vi "ATS_Buffer_to_Channel.vi"(8 "GetProcessedData":bool, 9 "MaxLength (-1)":i32=-1, 10 "Channel":T1, 11 "Buffer [AB]":u16[](array[numeric])) -> (2 "[B]":u16[](array[numeric]), 3 "[A]":u16[](array[numeric]))   [LabVIEW 2012]
doc: "_____AlazarTech, Scope_____\n\nExample to separate or Truncate Buffer data from ATS Async acquisition.\nHeader (if acquire) is include in data [A] and [B]."
uses:
  ATS_ctl/ATS_DMA_Channel.ctl
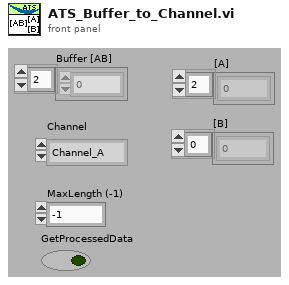
[diagram p1: front panel]
types:
  T1 = typedef "ATS_DMA_Channel.ctl" = enum16{"Channel_A", "Channel_B", "A & B"}
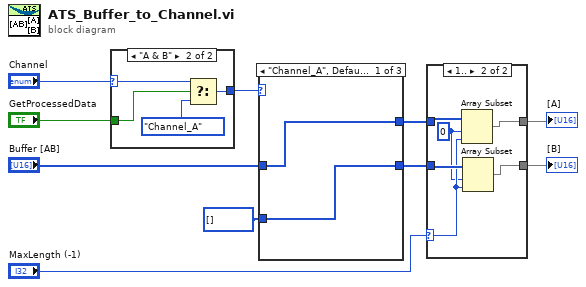
[diagram p0: block diagram]
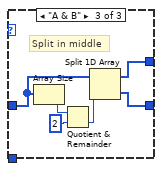
[diagram p5: hidden frame]
diagram:
  n1 = case shown="\"A & B\"" "Channel" {
    selector: "Channel" -> [w11 w12]
    tunnel: [w11 w15] -> w2
    tunnel: "GetProcessedData" -> [_ w14]
    frame "Channel_A", Default {
    }
    frame "A & B" {
      n2 = Select(t=w12, s=w14, f=ATS_DMA_Channel."Channel_A" ("t")) -> (s? t:f=w15:T1)
    }
  }
  n3 = case shown="\"Channel_A\", Default" w2 {
    tunnel: u16[] [] ("[B]") -> [w16 w18 _]
    tunnel: "Buffer [AB]" -> [w17 w19 w22]
    tunnel: [w16 w19 w20] -> w7
    tunnel: [w17 w18 w21] -> w5
    frame "Channel_A", Default {
    }
    frame "Channel_B" {
    }
    frame "A & B" {
      # "Split in middle"
      n4 = Array Size(array=w22) -> (size(s)=w25:i32)
      n5 = Quotient & Remainder(x=w25, y=2) -> (floor(x/y)=w23:i32)  [unwired: 1 out]
      n6 = Split 1D Array(array=w22, index=w23) -> (first subarray=w21:u16[], second subarray=w20:u16[])
    }
  }
  n7 = case shown="1.." "MaxLength (-1)" {
    selector: "MaxLength (-1)" -> [_ w29]
    tunnel: w7 -> [w27 w33]
    tunnel: [w27 w32] -> w6
    tunnel: w5 -> [w26 w31]
    tunnel: [w26 w30] -> w4
    frame ..0 {
    }
    frame 1.. {
      w28 = 0 ("index")
      n8 = Array Subset(array=w31, index=w28, length=w29) -> (w30:u16[])
      n9 = Array Subset(array=w33, index=w28, length=w29) -> (w32:u16[])
    }
  }
  "[A]" <- w4
  "[B]" <- w6
